vi "MatrixSwitchSingle.vi"(7 "Switch action":u16(ring) items=["Open", "Close"], 8 "error in (no error)":errorcluster, 9 "Matrix Y":i32=1 min=1 max=12 step=1, 10 "Matrix X":i32=1 min=1 max=12 step=1, 11 "GPIBSwitching in":refnum<class "GPIBSwitching.lvclass">) -> (0 "error out":errorcluster, 2 "command string":string, 3 "GPIBSwitching out":refnum<class "GPIBSwitching.lvclass">)   [LabVIEW 2018, in "GPIBSwitching.lvclass"]
uses:
  GPIBSwitching.lvclass
  C:/ProbeTestSoftware2019/itk-strip-sensor-qc/InstrControl/InstrControl.lvclass
  Matrix_CommandsGlobal.vi
  InstrControl.lvclass
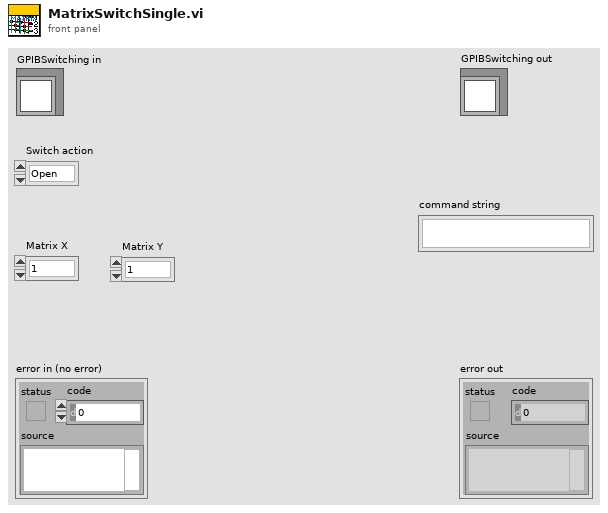
[diagram p1: front panel]
types:
  T1 = cluster{"Matrix address":string, "Instrument name":string, "Instrument type":u16, "Command \"Matrix Reset\"":string, "Command \"Connect Matrix Channels\"":string, "Command \"Disconnect Matrix Channels\"":string}
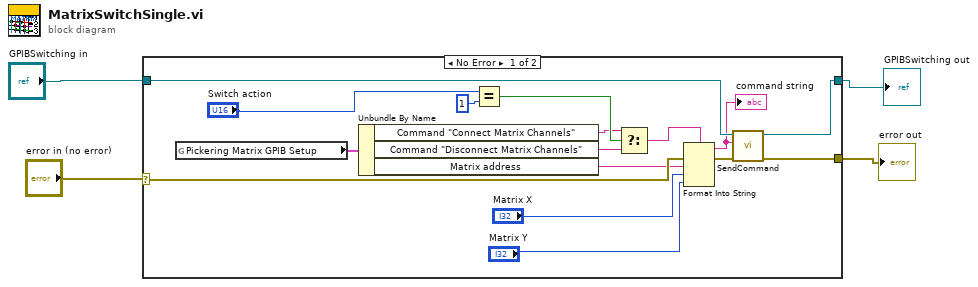
[diagram p0: block diagram]
diagram:
  n1 = case shown="No Error" "error in (no error)" {
    selector: "error in (no error)" -> [w20 w22]
    tunnel: [w17 w22] -> w2
    tunnel: [w16 w21] -> w1
    tunnel: "GPIBSwitching in" -> [w19 w21]
    frame No Error {
      n2 = global read "Matrix_CommandsGlobal.vi" "Pickering Matrix GPIB Setup"() -> (w15:T1)
      n3 = Unbundle By Name(w15) -> ("Command \"Connect Matrix Channels\""=w12:string, "Command \"Disconnect Matrix Channels\""=w11:string, "Matrix address"=w9:string)
      n4 = Equal?(x="Switch action", y=1) -> (x = y?=w13:bool)
      n5 = Select(t=w12, s=w13, f=w11) -> (s? t:f=w10:string)
      n6 = Format Into String(format string=w10, error in=w20, w9, "Matrix X", "Matrix Y") -> (resulting string=w7:string, error out=w18:errorcluster)  [unwired: 1 in]
      "command string" <- w7
      n7 = call "SendCommand.vi"("error in (no error)"=w18, "Command string"=w7, "InstControl in"=w19) -> ("error out"=w17:errorcluster, "InstControl out"=w16:refnum<class "GPIBSwitching.lvclass">)  [unwired: 7 in]
    }
    frame Error {
    }
  }
  "error out" <- w2
  "GPIBSwitching out" <- w1
